vi "Master on Desktop.vi"() -> ()   [LabVIEW 2021]
doc: "Demonstrates how to use Modbus functions to create a master communicating with a Modbus slave. It shows an interactive UI to allow users manually read and write the coils on the slave using TCP connection. Users can also change the timeout for reading operation if the network state is not good."
uses:
  API/Master/Modbus Master.lvclass/Modbus Master.ctl
  API/Wrapper/Create TCP Master.vi
  API/Master/Modbus Master.lvclass
  API/Wrapper/API Main.lvlib
panel:
  out "timer":u32(graph)
  in  "register values 2":u16[](array[numeric])
  out "register values":u16[](array[numeric])
  in  "Set Read Timeout":bool
  in  "Read Timeout (ms)":i32=5000
  in  "Read Count":u16=10
  in  "Stop":bool
  in  "Read":bool
  out "Coil Values Read":bool[](array[boolean])
  in  "Write":bool
  in  "Coil Values to Write":bool[](array[boolean])
  # "Overview: Demonstrates the use of the Modbus Master VIs to create a Modbus master and use the Modbus master to read and write coil values on a Modbus slave.\nRequirements: LabVIEW Datalogging and Supervisory Control Module\nInstructions:\n1. Ensure Slave On Desktop.vi is already running.\n2. Run the VI.\n3. Click Stop to stop the VI."
  # "Write Operation"
  # "Read Operation"
  # "Set Timeout For Read Operation"
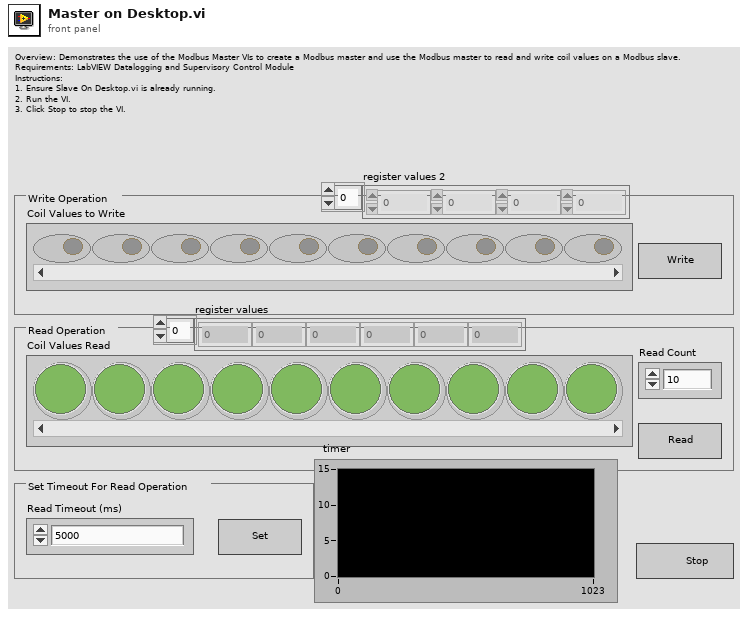
[diagram p1: front panel]
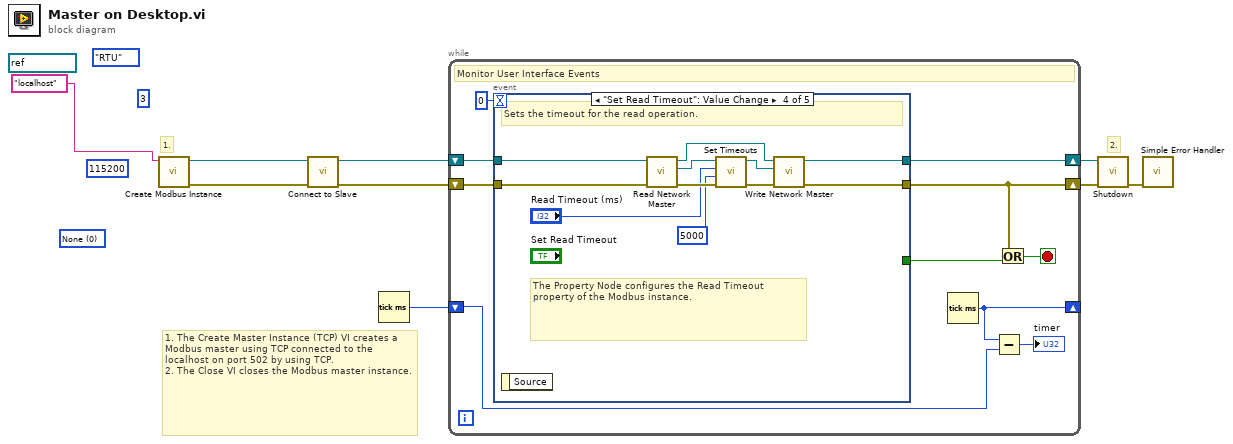
[diagram p0: block diagram]
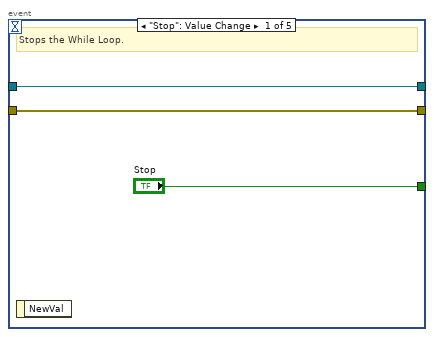
[diagram p2: hidden frame]
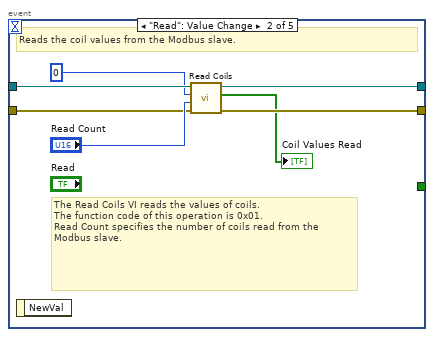
[diagram p3: hidden frame]
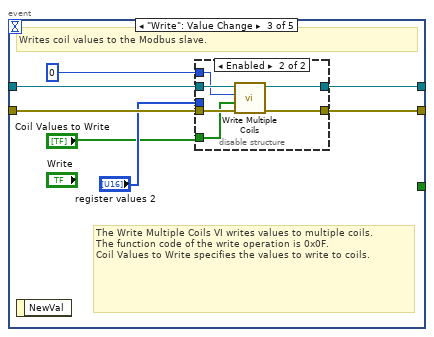
[diagram p4: hidden frame]
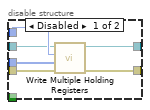
[diagram p5: hidden frame]
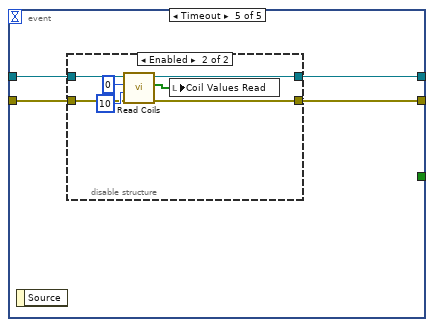
[diagram p6: hidden frame]
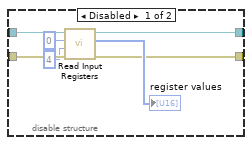
[diagram p7: hidden frame]
diagram:
  (unwired) refnum<visa-resource-name> "COM18" ("VISA resource name")
  (unwired) u16 0 items=["None", "Odd", "Even"] ("parity (Even)")
  (unwired) u32 115200 ("baud rate (9600)")
  (unwired) enum16{"RTU", "ASCII"}."RTU" ("serial type")
  (unwired) u8 3 ("unit ID")
  # "2."
  # "1."
  # "1. The Create Master Instance (TCP) VI creates a Modbus master using TCP connected to the localhost on port 502 by using TCP.\n2. The Close VI closes the Modbus master instance."
  n1 = call-poly "Create Modbus Instance.vi"("address"="localhost") -> ("error out"=w2:errorcluster, "TCP master instance"=w1:refnum<class "Modbus Master.lvclass">)  [unwired: 9 in]
  n2 = call-dynamic "Connect to Slave.vi"("error in (no error)"=w2, "Modbus master in"=w1) -> ("error out"=w6:errorcluster, "Modbus master out"=w3:refnum<class "Modbus Master.lvclass">)  [unwired: 8 in]
  n3 = Tick Count (ms)() -> (millisecond timer value=w5:u32)
  n4 = while {
    shift-right: [w18] -> w8
    shift-left: w3 -> [w19]
    shift-right: [w16] -> w9
    shift-left: w6 -> [w17]
    shift-right: [w11] -> _
    shift-left: w5 -> [w12]
    stop <- w14 stop-if-true
    # "Monitor User Interface Events"
    n5 = event shown="[3] \"Set Read Timeout\": Value Change" {
      selector: _ -> [_ _ _ _ _]
      dyn-events: _ -> [_ _ _ _ _]
      timeout: 0 -> [_ _ _ _ _]
      tunnel: ["Stop" _ _ _ _] -> w15
      tunnel: w19 -> [w21 w29 w35 w59 w63]
      tunnel: [w21 w28 w34 w50 w61] -> w18
      tunnel: w17 -> [w22 w25 w33 w57 w62]
      tunnel: [w22 w24 w32 w51 w60] -> w16
      event "Stop": Value Change {
        # "Stops the While Loop."
        n6 = event-data() -> ()  [unwired: 1 in, 1 out]
      }
      event "Read": Value Change {
        # "The Read Coils VI reads the values of coils.\nThe function code of this operation is 0x01.\nRead Count specifies the number of coils read from the Modbus slave."
        # "Reads the coil values from the Modbus slave."
        n7 = event-data() -> ()  [unwired: 1 in, 1 out]
        n8 = call-dynamic "Read Coils.vi"("error in (no error)"=w25, "number of coils"="Read Count", "starting address"=u16 0, "Modbus master in"=w29) -> ("error out"=w24:errorcluster, "coil values"=→"Coil Values Read":bool[], "Modbus master out"=w28:refnum<class "Modbus Master.lvclass">)  [unwired: 5 in]
      }
      event "Write": Value Change {
        # "The Write Multiple Coils VI writes values to multiple coils.\nThe function code of the write operation is 0x0F.\nCoil Values to Write specifies the values to write to coils."
        # "Writes coil values to the Modbus slave."
        n9 = event-data() -> ()  [unwired: 1 in, 1 out]
        n10 = disable-structure shown="Enabled" {
          disable-tunnel: u16 0 ("starting address") -> [w42 w43]
          disable-tunnel: w35 -> [w41 w48]
          disable-tunnel: [w40 w45] -> w34
          disable-tunnel: w33 -> [w39 w47]
          disable-tunnel: [w38 w46] -> w32
          disable-tunnel: "register values 2" -> [w37 _]
          disable-tunnel: "Coil Values to Write" -> [_ w44]
          frame Disabled {
            n11 = call-dynamic "Write Multiple Holding Registers.vi"("error in (no error)"=w39, "holding register values"=w37, "starting address"=w42, "Modbus master in"=w41) -> ("error out"=w38:errorcluster, "Modbus master out"=w40:refnum<class "Modbus Master.lvclass">)  [unwired: 6 in]
          }
          frame Enabled {
            n12 = call-dynamic "Write Multiple Coils.vi"("error in (no error)"=w47, "coil values"=w44, "starting address"=w43, "Modbus master in"=w48) -> ("error out"=w46:errorcluster, "Modbus master out"=w45:refnum<class "Modbus Master.lvclass">)  [unwired: 6 in]
          }
        }
      }
      event "Set Read Timeout": Value Change {
        # "The Property Node configures the Read Timeout property of the Modbus instance."
        # "Sets the timeout for the read operation."
        n13 = event-data() -> ()  [unwired: 1 in, 1 out]
        n14 = call "Read Network Master.vi"("error in"=w57, "Modbus master in"=w59) -> ("error out"=w56:errorcluster, "Network Master"=w58:refnum<class "Network Master.lvclass">, "Modbus master out"=w49:refnum<class "Modbus Master.lvclass">)  [unwired: 7 in]
        n15 = call "Set Timeouts.vi"("error in (no error)"=w56, "write operation timeout (ms)"=5000, "read operation timeout (ms)"="Read Timeout (ms)", "Modbus master in"=w58) -> ("error out"=w53:errorcluster, "Modbus master out"=w52:refnum<class "Network Master.lvclass">)  [unwired: 6 in]
        n16 = call "Write Network Master.vi"("error in"=w53, "Network Master"=w52, "Modbus master in"=w49) -> ("error out"=w51:errorcluster, "Modbus master out"=w50:refnum<class "Modbus Master.lvclass">)  [unwired: 7 in]
      }
      event Timeout {
        n17 = event-data() -> ()  [unwired: 1 in, 1 out]
        n18 = disable-structure shown="Enabled" {
          disable-tunnel: w63 -> [w70 w75]
          disable-tunnel: w62 -> [w69 w73]
          disable-tunnel: [w65 w74] -> w61
          disable-tunnel: [w64 w72] -> w60
          frame Disabled {
            n19 = call-dynamic "Read Input Registers.vi"("error in (no error)"=w69, "number of input registers"=u16 4 ("number of holding registers"), "starting address"=u16 0, "Modbus master in"=w70) -> ("error out"=w64:errorcluster, "register values"=→"register values":u16[], "Modbus master out"=w65:refnum<class "Modbus Master.lvclass">)  [unwired: 5 in]
          }
          frame Enabled {
            n20 = call-dynamic "Read Coils.vi"("error in (no error)"=w73, "number of coils"=u16 10 ("number of holding registers"), "starting address"=u16 0, "Modbus master in"=w75) -> ("error out"=w72:errorcluster, "coil values"=w71:bool[], "Modbus master out"=w74:refnum<class "Modbus Master.lvclass">)  [unwired: 5 in]
            n21 = local write "Coil Values Read"(w71) -> ()
          }
        }
      }
    }
    n22 = Tick Count (ms)() -> (millisecond timer value=w11:u32)
    n23 = Subtract(x=w11, y=w12) -> (x-y=→"timer":u32)
    n24 = Or(x=w16, y=w15) -> (x .or. y?=w14:bool)
  }
  n25 = call-dynamic "Shutdown.vi"("error in (no error)"=w9, "Modbus master in"=w8) -> ("error out"=w7:errorcluster)  [unwired: 9 in]
  n26 = call <vilib>:"Simple Error Handler.vi"("error in (no error)"=w7) -> ()  [unwired: 4 in, 5 out]
